vi "InitInstrument.vi"(8 "error in (no error)":errorcluster, 11 "wAddress":i16) -> (0 "error out":errorcluster, 3 "function return":i16)   [LabVIEW 2013, in "HS3OverallRoutines.lvlib"]
doc: "Descriptions: Initialize the hardware of the instrument. Set default measurementsettings, allocate memory and obtain the calibration constants etc. Parallel port connected instruments, USB instruments and PCI bus instruments detect the hardware by themselves and ignore the address parameters.\n\nInput: wAddress The hardware address of the instrument should be passed to this routine.\nOutput: Return value E_NO_ERRORS | E_NO_HARDWARE\n\nFunction prototype: word InitInstrument( word wAddress )\n\nshort int InitInstrument ( short int wAddress );"
uses:
  HS3OverallRoutines.lvlib
  hs3.dll
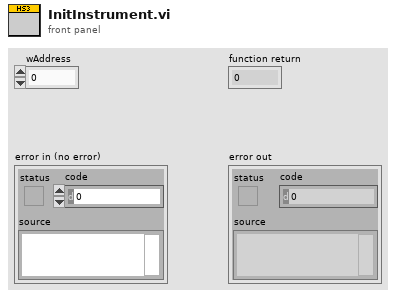
[diagram p1: front panel]
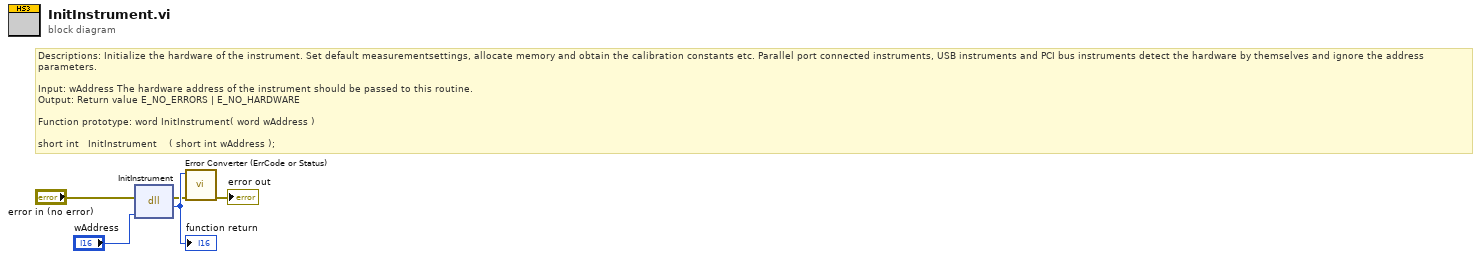
[diagram p0: block diagram]
diagram:
  # "Descriptions: Initialize the hardware of the instrument. Set default measurementsettings, allocate memory and obtain the calibration constants etc. Parallel port connected instruments, USB instruments and PCI bus instruments detect the hardware by themselves and ignore the address parameters.\n\nInput: wAddress The hardware address of the instrument should be passed to this routine.\nOutput: Return value E_NO_ERRORS | E_NO_HARDWARE\n\nFunction prototype: word InitInstrument( word wAddress )\n\nshort int \t\tInitInstrument\t\t\t\t( short int wAddress );"
  n1 = dll-call lib="C:/Documents and Settings/admin/Pulpit/HS3 LabViewLib/HS3_WRAPPER/OverallRoutines/hs3.*" fn="InitInstrument"(error in="error in (no error)", "wAddress"="wAddress") -> (error out=w2:errorcluster, w5:i16)  [unwired: 3 in, 1 out]
  "function return" <- w5
  n2 = call "Error Converter (ErrCode or Status).vi"("error in (no error)"=w2, "error code"=w5) -> ("error out"=→"error out":errorcluster)  [unwired: 9 in]
